vi "Ignore Error.vi"(8 "error in":errorcluster, 11 "Error Code":i32) -> (0 "error out":errorcluster)   [LabVIEW 2013, in "LVTM.lvlib"]
uses:
  LVTM.lvlib
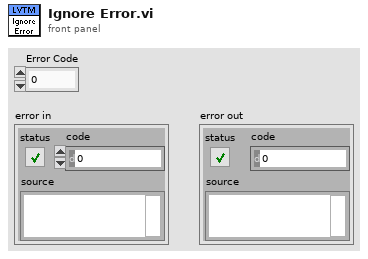
[diagram p1: front panel]
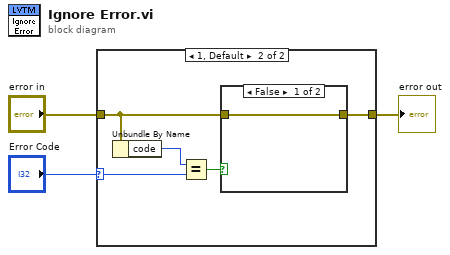
[diagram p0: block diagram]
diagram:
  n1 = case shown="1, Default" "Error Code" {
    selector: "Error Code" -> [_ w5]
    tunnel: "error in" -> [w4 w9]
    tunnel: [w4 w8] -> w2
    frame 0 {
    }
    frame 1, Default {
      n2 = Unbundle By Name(w9) -> ("code"=w6:i32)
      n3 = Equal?(x=w6, y=w5) -> (x = y?=w7:bool)
      n4 = case shown="False" w7 {
        tunnel: [w10 _] -> w8
        tunnel: w9 -> [w10 _]
        frame False {
        }
        frame True {
        }
      }
    }
  }
  "error out" <- w2
